vi "Check and save IG.vi"(1 "IG save time (s)":i32=90, 2 "Time Since Last Shot":dbl=186.99969625473022 step=8.0 format="%<%H:%M:%S>t", 3 "name or relative path":string="IG1vsTimeNew.csv", 4 "error in":errorcluster, 5 "LatestShotNetworkPath":path=path "\\\\polaris\\SPECTOR Data/015567", 6 "Last Shot Save Path":path=path "C:/Data/LocalDataSPECTOR1/015567", 7 "IGvsTime Array":dbl[][](array[numeric])=[[3576160860.5582724, 1.7450302828254615e-08], [3576160861.5493293, 1.7268046680150338e-08], [3576160862.5563865, 1.73589355612912e-08], [3576160863.5474434, 1.7542150998983254e-08], [3576160864.554501, 1.7450302828254615e-08], [3576160865.5615587, 1.7450302828254615e-08], [3576160866.552615, 1.73589355612912e-08], [3576160867.558673, 1.7634482604672875e-08], [3576160868.5497293, 1.7634482604672875e-08], [3576160869.556787, 1.7542150998983254e-08], [3576160870.547844, 1.7634482604672875e-08], [3576160871.5389004, 1.772730018984185e-08], [3576160872.560959, 1.7634482604672875e-08], [3576160873.5360146, 1.7542150998983254e-08], [3576160874.543072, 1.7450302828254615e-08], [3576160875.534129, 1.7542150998983254e-08], [3576160876.541187, 1.7542150998983254e-08], [3576160877.548244, 1.7634482604672875e-08], [3576160878.538301, 1.772730018984185e-08], [3576160879.545358, 1.7542150998983254e-08], [3576160880.536415, 1.7634482604672875e-08], [3576160881.543473, 1.7634482604672875e-08], [3576160882.534529, 1.7542150998983254e-08], [3576160883.541587, 1.7634482604672875e-08], [3576160884.5476446, 1.7634482604672875e-08], [3576160885.538701, 1.7634482604672875e-08], [3576160886.5457587, 1.7542150998983254e-08], [3576160887.5368156, 1.7634482604672875e-08], [3576160888.5438733, 1.7542150998983254e-08], [3576160889.5659313, 1.7634482604672875e-08], [3576160890.5569882, 1.7634482604672875e-08], [3576160891.564046, 1.7634482604672875e-08], [3576160892.5551023, 1.7634482604672875e-08], [3576160893.56216, 1.7634482604672875e-08], [3576160894.5682178, 1.7634482604672875e-08], [3576160895.559274, 1.7634482604672875e-08], [3576160896.566332, 1.7634482604672875e-08], [3576160897.557389, 1.7634482604672875e-08], [3576160898.548445, 1.7634482604672875e-08], [3576160899.539502, 1.7634482604672875e-08], [3576160900.5455594, 1.7820606312401403e-08], [3576160901.552617, 1.772730018984185e-08], [3576160902.543674, 1.7634482604672875e-08], [3576160903.550731, 1.772730018984185e-08], [3576160904.541788, 1.772730018984185e-08], [3576160905.547846, 1.7820606312401403e-08], [3576160906.5549035, 1.772730018984185e-08], [3576160907.54596, 1.73589355612912e-08], [3576160947.565249, 2.064234498888727e-08], [3576160948.5563054, 1.6044453761858692e-08], [3576160949.563363, 1.546556522750193e-08], [3576160950.5534196, 1.6557859686369703e-08], [3576160951.5604773, 1.8294555459365935e-08], [3576160952.551534, 1.9382085632218174e-08], [3576160953.558592, 1.9382085632218174e-08], [3576160954.5656495, 1.8879962310764135e-08], [3576160955.556706, 1.8390847281334535e-08], [3576160956.5637636, 1.8294555459365935e-08], [3576160957.55382, 1.8294555459365935e-08], [3576160958.560878, 1.8487645927040906e-08], [3576160959.5679355, 1.8584954064108234e-08], [3576160960.558992, 1.8487645927040906e-08], [3576160961.5660496, 1.8487645927040906e-08], [3576160962.556106, 1.8390847281334535e-08], [3576160963.5631638, 1.8294555459365935e-08], [3576160964.5702214, 1.8294555459365935e-08], [3576160965.5612783, 1.819876780747909e-08], [3576160966.568336, 1.819876780747909e-08], [3576160967.5583925, 1.8103481685912254e-08], [3576160968.56545, 1.8103481685912254e-08], [3576160969.5565066, 1.8103481685912254e-08], [3576160970.5635643, 1.8103481685912254e-08], [3576160971.570622, 1.8103481685912254e-08], [3576160972.5616784, 1.8008694468725098e-08], [3576160973.568736, 1.7914403543726225e-08], [3576160974.574794, 1.8103481685912254e-08], [3576160975.5818515, 1.8008694468725098e-08], [3576160976.588909, 1.8008694468725098e-08], [3576160977.5799656, 1.7914403543726225e-08], [3576160978.5870233, 1.7820606312401403e-08], [3576160979.5780797, 1.772730018984185e-08], [3576160980.5681367, 1.7634482604672875e-08], [3576160981.559193, 1.7542150998983254e-08], [3576160982.55025, 1.7542150998983254e-08], [3576160983.5573077, 1.7634482604672875e-08], [3576160984.548364, 1.772730018984185e-08], [3576160985.554422, 1.772730018984185e-08], [3576160986.5454783, 1.7634482604672875e-08], [3576160987.552536, 1.772730018984185e-08], [3576160988.5595937, 1.772730018984185e-08], [3576160989.55065, 1.772730018984185e-08], [3576160990.557708, 1.7820606312401403e-08], [3576160991.5487647, 1.7820606312401403e-08], [3576160992.554822, 1.7820606312401403e-08], [3576160993.5618796, 1.772730018984185e-08], [3576160994.5529366, 1.772730018984185e-08], [3576160995.559994, 1.7820606312401403e-08], [3576160996.5510507, 1.7820606312401403e-08], [3576160997.5581083, 1.8008694468725098e-08], [3576160998.548165, 1.7914403543726225e-08], [3576160999.5552225, 1.7820606312401403e-08], [3576161000.56228, 1.772730018984185e-08], [3576161001.553337, 1.7820606312401403e-08], [3576161002.5603943, 1.772730018984185e-08], [3576161003.5504513, 1.7914403543726225e-08], [3576161004.5575085, 1.772730018984185e-08], [3576161005.5485654, 1.772730018984185e-08], [3576161006.555623, 1.8103481685912254e-08], [3576161007.5626807, 1.819876780747909e-08], [3576161008.553737, 1.819876780747909e-08], [3576161009.560795, 1.819876780747909e-08], [3576161010.5508513, 1.819876780747909e-08], [3576161011.557909, 1.819876780747909e-08], [3576161012.5649667, 1.819876780747909e-08], [3576161013.5560236, 1.7914403543726225e-08], [3576161014.563081, 1.8103481685912254e-08], [3576161015.553138, 1.7634482604672875e-08], [3576161016.576196, 1.7820606312401403e-08], [3576161017.583254, 1.8008694468725098e-08], [3576161018.5743103, 1.8294555459365935e-08], [3576161019.580368, 1.8103481685912254e-08], [3576161020.5714245, 1.8008694468725098e-08], [3576161021.578482, 1.8103481685912254e-08], [3576161022.569539, 1.8103481685912254e-08], [3576161023.5765967, 1.8103481685912254e-08], [3576161024.583654, 1.8103481685912254e-08], [3576161025.573711, 1.8103481685912254e-08], [3576161026.580768, 1.8103481685912254e-08], [3576161027.571825, 1.8103481685912254e-08], [3576161028.5788827, 1.819876780747909e-08], [3576161029.5859404, 1.8294555459365935e-08], [3576161030.576997, 1.819876780747909e-08], [3576161031.5830545, 1.819876780747909e-08], [3576161032.574111, 1.8103481685912254e-08], [3576161033.565168, 1.8294555459365935e-08], [3576161034.5882263, 1.8103481685912254e-08], [3576161035.578283, 1.819876780747909e-08], [3576161036.5693398, 1.8294555459365935e-08], [3576161037.5763974, 1.819876780747909e-08], [3576161038.567454, 1.8008694468725098e-08], [3576161039.558511, 1.8103481685912254e-08], [3576161040.549567, 1.8103481685912254e-08], [3576161041.556625, 1.8103481685912254e-08], [3576161042.547682, 1.8294555459365935e-08], [3576161043.553739, 1.819876780747909e-08], [3576161044.544796, 1.819876780747909e-08], [3576161045.551853, 1.8390847281334535e-08], [3576161046.558911, 1.8103481685912254e-08], [3576161047.549968, 1.7820606312401403e-08], [3576161048.5570254, 1.7820606312401403e-08], [3576161049.547082, 1.7914403543726225e-08], [3576161050.5541396, 1.8008694468725098e-08], [3576161051.545196, 1.8103481685912254e-08], [3576161052.5522537, 1.8103481685912254e-08], [3576161053.5583115, 1.8103481685912254e-08], [3576161054.549368, 1.8103481685912254e-08], [3576161055.5564256, 1.8103481685912254e-08], [3576161056.5474825, 1.8008694468725098e-08], [3576161057.570541, 1.819876780747909e-08], [3576161058.5775986, 1.819876780747909e-08], [3576161059.5516543, 1.819876780747909e-08], [3576161060.5747128, 1.8103481685912254e-08], [3576161061.5497684, 1.8103481685912254e-08], [3576161062.556826, 1.8008694468725098e-08], [3576161063.5478826, 1.8103481685912254e-08], [3576161064.5539403, 1.8103481685912254e-08], [3576161065.560998, 1.8103481685912254e-08], [3576161066.5520544, 1.8103481685912254e-08], [3576161067.559112, 1.8103481685912254e-08], [3576161068.550169, 1.8103481685912254e-08], [3576161069.5562263, 1.819876780747909e-08], [3576161070.563284, 1.8103481685912254e-08], [3576161071.554341, 1.8103481685912254e-08], [3576161072.5613985, 1.8008694468725098e-08], [3576161073.551455, 1.8103481685912254e-08], [3576161074.5585127, 1.8103481685912254e-08], [3576161075.549569, 1.8103481685912254e-08], [3576161076.556627, 1.8103481685912254e-08], [3576161077.5636845, 1.819876780747909e-08], [3576161078.554741, 1.819876780747909e-08], [3576161079.5607986, 1.8103481685912254e-08], [3576161080.551855, 1.819876780747909e-08], [3576161081.5589128, 1.8008694468725098e-08], [3576161082.5659704, 1.8008694468725098e-08], [3576161083.5570273, 1.8103481685912254e-08], [3576161084.564085, 1.8008694468725098e-08], [3576161085.5541415, 1.8008694468725098e-08], [3576161086.561199, 1.7914403543726225e-08], [3576161087.5682564, 1.8103481685912254e-08], [3576161088.5593133, 1.7914403543726225e-08], [3576161089.566371, 1.8008694468725098e-08], [3576161090.5564275, 1.8008694468725098e-08], [3576161091.563485, 1.819876780747909e-08], [3576161092.5545416, 1.8103481685912254e-08], [3576161093.5455985, 1.8103481685912254e-08]]) -> (0 "error out":errorcluster)   [LabVIEW 2016]
uses:
  <vilib>/Utility/file.llb/Write To Spreadsheet File (DBL).vi
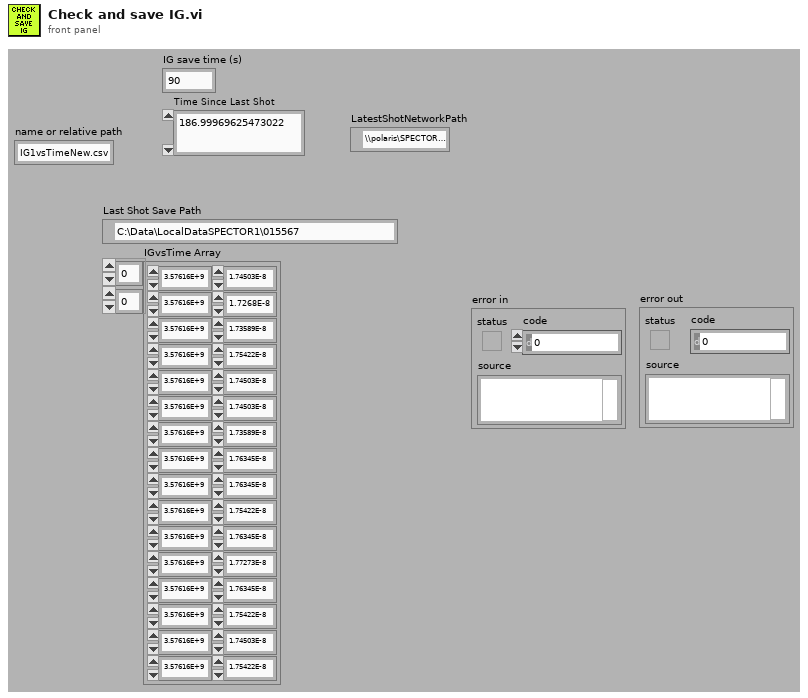
[diagram p1: front panel]
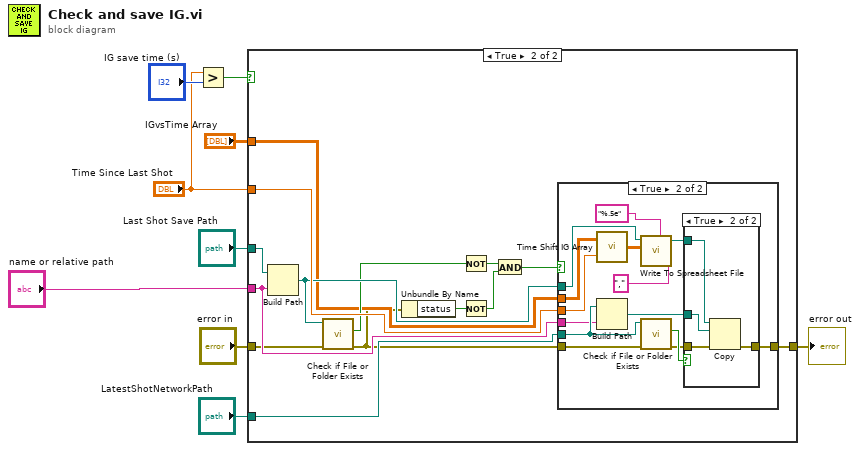
[diagram p0: block diagram]
diagram:
  n1 = Greater?(x="Time Since Last Shot", y="IG save time (s)") -> (0:w9:bool)
  n2 = case shown="True" w9 {
    tunnel: "Time Since Last Shot" -> [_ w24]
    tunnel: "Last Shot Save Path" -> [_ w17]
    tunnel: "IGvsTime Array" -> [_ w16]
    tunnel: "LatestShotNetworkPath" -> [_ w15]
    tunnel: "name or relative path" -> [_ w14]
    tunnel: [w10 w12] -> w2
    tunnel: "error in" -> [w10 w11]
    frame False {
    }
    frame True {
      n3 = Build Path(base path=w17, name or relative path=w14) -> (appended path=w23:path)
      n4 = call <vilib>:"Check if File or Folder Exists.vi"("error in (no error)"=w11, "path"=w23) -> ("error out"=w13:errorcluster, "file or folder exists?"=w21:bool)  [unwired: 7 in, 1 out]
      n5 = Unbundle By Name(w13) -> ("status"=w20:bool)
      n6 = Not(x=w21) -> (.not. x?=w18:bool)
      n7 = Not(x=w20) -> (.not. x?=w19:bool)
      n8 = And(x=w18, y=w19) -> (x .and. y?=w22:bool)
      n9 = case shown="True" w22 {
        tunnel: w24 -> [_ w39]
        tunnel: w23 -> [_ w35]
        tunnel: w16 -> [_ w31]
        tunnel: w15 -> [_ w30]
        tunnel: w14 -> [_ w29]
        tunnel: w13 -> [w25 w28]
        tunnel: [w25 w26] -> w12
        frame False {
        }
        frame True {
          n10 = call "Time Shift IG Array.vi"("Time Since Last Shot"=w39, "IGvsTime Array"=w31) -> ("IGvsTime TimeShifted"=w36:dbl[][])
          n11 = Build Path(base path=w30, name or relative path=w29) -> (appended path=w32:path)
          n12 = call-poly <vilib>:"Write To Spreadsheet File.vi"("delimiter (\\t)"="," ("delimiter (\\t)"), "format (%.3f)"="%.5e", "2D data"=w36, "file path (dialog if empty)"=w35) -> ("new file path (Not A Path if cancelled)"=w33:path)  [unwired: 4 in]
          n13 = call <vilib>:"Check if File or Folder Exists.vi"("error in (no error)"=w28, "path"=w30) -> ("error out"=w27:errorcluster, "file or folder exists?"=w34:bool)  [unwired: 7 in, 1 out]
          n14 = case shown="True" w34 {
            tunnel: w33 -> [_ w44]
            tunnel: w32 -> [_ w43]
            tunnel: w27 -> [w40 w42]
            tunnel: [w40 w41] -> w26
            frame False {
            }
            frame True {
              n15 = Copy(8:w42, 10:w43, 11:w44) -> (0:w41:errorcluster)  [unwired: 2 in, 2 out]
            }
          }
        }
      }
    }
  }
  "error out" <- w2
